vi "cooked.vi"(10 "destination":cluster{dbl, dbl, dbl}, 11 "current":T1) -> (3 "Numeric":dbl)   [LabVIEW 2017]
uses:
  040-typeDefs/Position.ctl
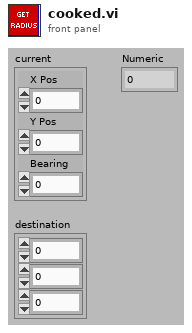
[diagram p1: front panel]
types:
  T1 = typedef "Position.ctl" = cluster{"X Pos":dbl, "Y Pos":dbl, "Bearing":dbl}
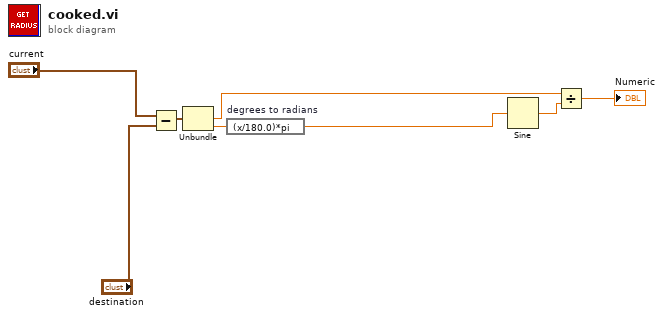
[diagram p0: block diagram]
diagram:
  n1 = Subtract(x="current", y="destination") -> (x-y=w3:T1)
  n2 = Unbundle(w3) -> ("Y Pos"=w6:dbl, "Bearing"=w4:dbl)  [unwired: 1 out]
  n3 = expression code="(x/180.0)*pi" "degrees to radians"(w4) -> (w5:dbl)
  n4 = Sine(x=w5) -> (sin(x)=w7:dbl)
  n5 = Divide(x=w6, y=w7) -> (x/y=→"Numeric":dbl)
